vi "EMG.vi"() -> ()   [LabVIEW 2019]
uses:
  <vilib>/addons/Biomedical/Biosignal Measurements/Biosignal Preprocessing/Biosignal RMS (Waveform).vi
  <vilib>/addons/Biomedical/NI_BMTK_Measurements.lvlib
panel:
  out "RMS":waveform(dbl)(graph)
  out "EMG":dynamicdata(graph)
  in  "stop":bool
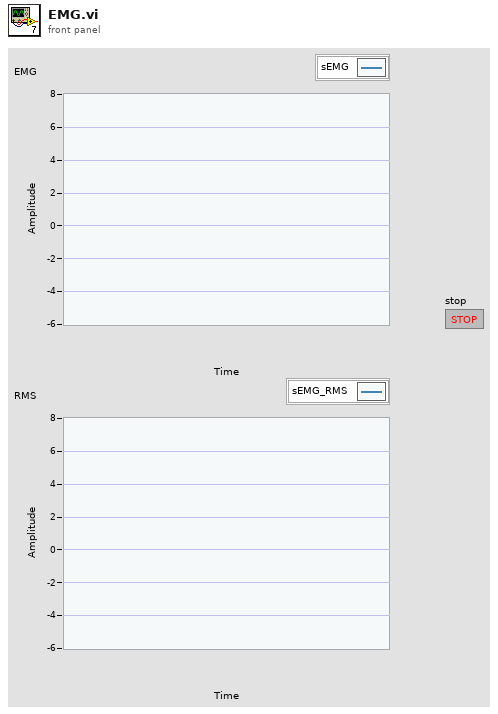
[diagram p1: front panel]
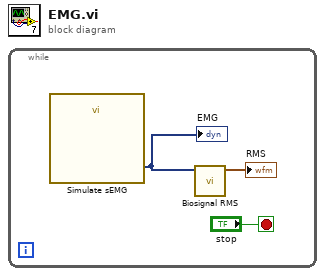
[diagram p0: block diagram]
diagram:
  n1 = while {
    stop <- "stop" stop-if-true
    n2 = call "Simulate sEMG"() -> ("EMG"=w2:dynamicdata)  [unwired: 10 in, 1 out]
    "EMG" <- w2
    n3 = call-poly <vilib>:"Biosignal RMS.vi"("biosignal"=w2) -> ("RMS value"=→"RMS":waveform(dbl))  [unwired: 9 in, 1 out]
  }
